vi "readFromXML.vi"(8 "error in (no error)":errorcluster, 10 "XMLin":string, 11 "TCSIersCommand in":refnum<class "TCSIersCommand.lvclass">) -> (0 "error out":errorcluster, 3 "TCSIersCommand out":refnum<class "TCSIersCommand.lvclass">)   [LabVIEW 2022 SP3, in "TCSDataDefinitions.lvlib" / "TCSTimeComponentCommand.lvlib" / "TCSIersCommand.lvclass"]
uses:
  TCSIersCommand.lvclass
  TCSCommand/TCSCommand/TCSCommand.lvclass
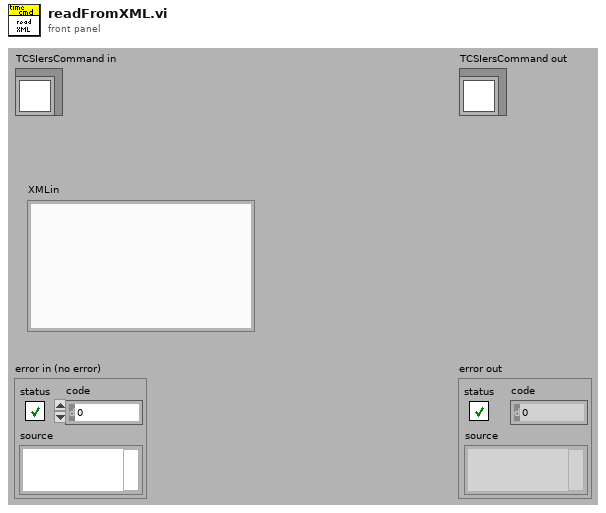
[diagram p1: front panel]
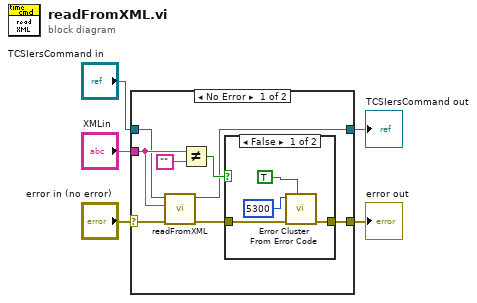
[diagram p0: block diagram]
diagram:
  n1 = case shown="No Error" "error in (no error)" {
    selector: "error in (no error)" -> [w9 w20]
    tunnel: [w11 w20] -> w4
    tunnel: [w6 w19] -> w2
    tunnel: "TCSIersCommand in" -> [w7 w19]
    tunnel: "XMLin" -> [w10 _]
    frame No Error {
      n2 = call-parent "readFromXML.vi"("error in (no error)"=w9, "XML in"=w10, "TCSCommand in"=w7) -> ("error out"=w8:errorcluster, "TCSCommand out"=w6:refnum<class "TCSIersCommand.lvclass">)  [unwired: 7 in]
      n3 = Not Equal?(x=w10, y="") -> (x != y?=w12:bool)
      n4 = case shown="False" w12 {
        tunnel: [w15 w18] -> w11
        tunnel: w8 -> [w16 w18]
        frame False {
          n5 = call <vilib>:"Error Cluster From Error Code.vi"("show call chain? (False)"=TRUE, "error in (no error)"=w16, "error code (0)"=5300 ("code")) -> ("error out"=w15:errorcluster)  [unwired: 6 in]
        }
        frame True {
        }
      }
    }
    frame Error {
    }
  }
  "error out" <- w4
  "TCSIersCommand out" <- w2
